vi "_[error50004]Add Tag After Locking.vi"(8 "error in (no error)":errorcluster, 9 "db name":string, 10 "tag name":string) -> (0 "error out":errorcluster)   [LabVIEW 2017, in "TagDB(DEV).lvlib"]
uses:
  TagDB(DEV).lvlib
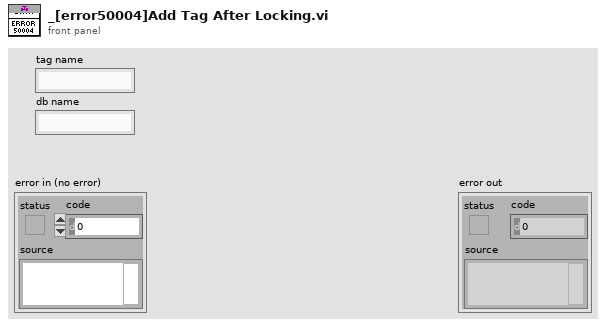
[diagram p1: front panel]
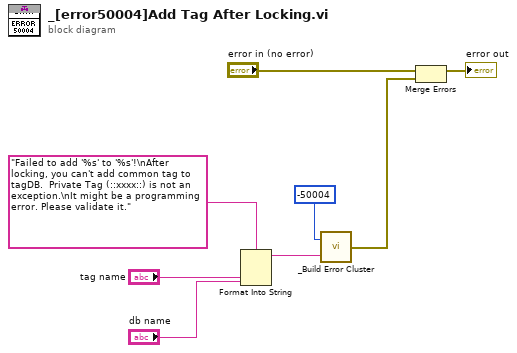
[diagram p0: block diagram]
diagram:
  n1 = Format Into String(format string="Failed to add '%s' to '%s'!\nAfter locking, you can't add common tag to tagDB.  Private Tag (::xxxx::) is not an exception.\nIt might be a programming error. Please validate it." ("source"), "tag name", "db name") -> (resulting string=w2:string)  [unwired: 2 in, 1 out]
  n2 = call "_Build Error Cluster.vi"("String to Prepend to source (\"\")"=w2, "code"=-50004) -> ("error out"=w1:errorcluster)
  n3 = Merge Errors("error in (no error)", w1) -> (→"error out":errorcluster)
